vi "Multirecord Acquisition FPGA_20221228.vi"() -> ()   [LabVIEW 2021]
doc: "Use this VI as a template for the reconfigurable oscilloscope acquisition design. The block diagram is divided into three main loops.\n\nRegister Bus: This loop initializes the registers that are needed to support the configuration of the device. The FIFO bus, on the left, allows all the other design libraries to communicate with one another. This loop is very important to support the proper behavior of the instrument design library components.\n\nAcquisition: Acquires data from the I/O channels and writes the data into the record memory using the <B>Write</B> VI of the Multirecord Acquisition instrument design library. This VI also evaluates the various acquisition triggers and decides whether to acquire each data value in record memory. The host level VI (Fetch Record.vi) can read acquired records from the DRAM. The data is stored in 2 DRAM banks, each with 768 MB of storage.\n\nFetch: The recorded data is retrieved when the <B>Fetch Single Record</B> VI is run from the host VI. The <B>Write to Fetch DMA FIFO</B> VI writes data to the acq.fetch fifo 0 to transmit record data form the FPGA to the record fetch VIs on the host. This DMA FIFO must have a predefined name based on the instance parameter. By default, it is 0 (since the associated terminal on the <B>Create Resources DRAM Write Read</B> VI is unwired), so the connected FIFO is named acq.fetch fifo 0."
uses:
  FPGA Interface Typedefinitions/Trigger Combination Type.ctl
  Host/Clusts/AllWindowsClust.ctl
  Host/Clusts/ChannelWindowClust.ctl
  Controls/Clust/WindowTriggerClust.ctl
  <instrlib>/_niInstr/Data Trigger/v1/Shared/Public/Level Configuration FXP(+-,18,1).ctl
  <instrlib>/_niInstr/Data Trigger/v1/Shared/Public/Level Configuration Trigger When.ctl
  <vilib>/Platform/TimedLoop/XDataNode/timing_clust.ctl
  <vilib>/Platform/TimedLoop/XDataNode/nitl_modes.ctl
  <vilib>/Platform/TimedLoop/XDataNode/wakeup.ctl
  Controls/Clust/All_acquisition_Resources.ctl
  <instrlib>/_niInstr/Multirecord Acquisition/Common/v1/FPGA/niInstr Multirecord Acquisition Common v1 FPGA.lvclass
  C:/Program Files (x86)/National Instruments/LabVIEW 2021/instr.lib/_niInstr/Multirecord Acquisition/Interface/v1/FPGA/niInstr Multirecord Acquisition v1 FPGA.lvclass
  Trigger/SubVIs/Types/Trigger Type.ctl
  <instrlib>/_niInstr/Data Trigger/v1/Shared/Public/Edge Configuration FXP(+-,18,1).ctl
  <instrlib>/_niInstr/Data Trigger/v1/Shared/Public/Edge Configuration Trigger Slope.ctl
  Controls/Clust/Update_Trigger_Center.ctl
  Controls/Clust/Status_Booleans_Clust.ctl
  Controls/Clust/Trig_Config_Clust.ctl
  <instrlib>/_niInstr/FIFO Register Bus/v1/FPGA/niInstr FIFO Register Bus v1 FPGA.lvclass
  C:/Program Files (x86)/National Instruments/LabVIEW 2021/instr.lib/_niInstr/Instruction Framework/v1/FPGA/Interfaces/Instruction Producer/Instruction Producer.lvclass
  <vilib>/rvi/Emulation/niFpgaSctlEmulationGetInTimedLoop.vi
  <vilib>/rvi/Emulation/niFpgaEmulationReportErrorSimple.vi
  <vilib>/rvi/Emulation/niFpgaGetClockAttributes.vi
  <vilib>/rvi/Emulation/niFpgaCriticalErrorInLSC.vi
  <instrlib>/_niInstr/Multirecord Acquisition/Common/v1/FPGA/Private/Create Fetch DMA FIFO Resources U8x32.vi
  <instrlib>/_niInstr/Multirecord Acquisition/Common/v1/FPGA/Private/Create Resources DRAM U384x2 U768 Write Read.vi
  <instrlib>/_niInstr/Basic Elements/v1/FPGA/Private/Count Up U32.vi
  <vilib>/rvi/eio/common/nirviEmuTemplateMethod_errors.vi
  <instrlib>/HSAI-RIO/Config/Group A/v1/FPGA/Digital Correction/Validate 8 Channel Data.vi
  <instrlib>/HSAI-RIO/Config/Group A/v1/FPGA/Digital Correction/Digital Correction (8 Ch).vi
  <instrlib>/HSAI-RIO/Config/Group A/v1/FPGA/Digital Correction/FIR Filter (8 Ch).vi
  DSP/SubVIs/Integer decimationx8ch.vi
  Data Type Conversion/SubVIs/Remove Overflow FXP(+-,18,1)x8ch.vi
  Trigger/Trigger FXP(+,-,18,1).vi
  Data Type Conversion/SubVIs/Data Type Conversion FXP(+-,18,1) to I16x8ch.vi
  <instrlib>/_niInstr/Channel/v1/FPGA/Private/Select and Interleave/Select And Interleave I16xNspcx8ch.vi
  <instrlib>/_niInstr/Multirecord Acquisition/Interface/v1/FPGA/Private/Write I16 Wrapper.vi
  <instrlib>/_niInstr/Multirecord Acquisition/Interface/v1/FPGA/Private/Retrieve Record U16 Wrapper.vi
  <instrlib>/_niInstr/Multirecord Acquisition/Interface/v1/FPGA/Private/Write to Fetch DMA FIFO U16 Wrapper.vi
  <vilib>/Platform/TimedLoop/XDataNode/XDataNode.xnode
  <vilib>/eio/EIONode/EIONode.xnode
  <instrlib>/_niInstr/Instruction Framework/v1/FPGA/Top Level Bus/Register Configuration/Register Configuration.lvclass
  <vilib>/Platform/TimedLoop/XDataNode/XDNodeRunTimeDep.lvlib
  <instrlib>/_niInstr/Multirecord Acquisition/Interface/v1/FPGA/niInstr Multirecord Acquisition v1 FPGA.lvclass
  <vilib>/rvi/LocalResourceManager/LocalResourceManager.xnode
  <vilib>/rvi/eio/common/nirviEmuReportErrorAndStop.vi
  <vilib>/rvi/DataTransferAndStorage/Container/Common/niFpgaContainerGetUniqueNameForEmu.vi
  <vilib>/rvi/DataTransferAndStorage/Container/Common/niFpgaContainerSetEmuInfo.vi
  <instrlib>/_niInstr/Channel/v1/FPGA/niInstr Channel v1 FPGA.lvlib
  <instrlib>/_niInstr/Basic Elements/v1/FPGA/niInstr Basic Elements v1 FPGA.lvlib
  <instrlib>/HSAI-RIO/Config/Group A/v1/FPGA/Digital Correction/Digital Correction.lvclass
  <instrlib>/HSAI-RIO/Config/Group A/v1/FPGA/Config Registers/Config Registers.lvclass
  <instrlib>/_niInstr/Data Trigger/v1/Shared/niInstr Data Trigger v1 Shared.lvlib
  Emulation/SubVIs/2 Element Generate Sine Cos Data FXP(+,-,14,1).vi
  <instrlib>/_niInstr/Multirecord Acquisition/Common/v1/FPGA/Private/Create Resources DRAM U384.vi
  <instrlib>/_niInstr/Multirecord Acquisition/Common/v1/FPGA/Private/Create Resources BRAM U384.vi
  <instrlib>/_niInstr/Multirecord Acquisition/Common/v1/FPGA/Private/Create Resources BRAM U768.vi
  FPGA Interface Typedefinitions/FPGA Interface Typedefinitions.lvlib
  C:/Program Files (x86)/National Instruments/LabVIEW 2021/instr.lib/_niInstr/Multirecord Acquisition/Common/v1/FPGA/niInstr Multirecord Acquisition Common v1 FPGA.lvclass
panel:
  out "Trigger Index":u16
  out "TrigCount":u32
  out "TrigCfg 0":T1
  in  "ResetTrig":bool
  in  "UserTrig":T4
  in  "trigger.rearm delay":u16=2
  in  "start trigger":bool=TRUE
  in  "reset":bool
  in  "trigger.combination type":T6
  out "fifo reg bus data 0":u64
  out "fifo reg bus status 0":u32
  in  "fifo reg bus ctrl 0":u32
  out "overflow":bool
  in  "dsp.decimation factor":u16
  out "overload":bool
  # "Register Bus Controls"
  # "FPGA"
  # "Acquisition Loop Controls"
  # "DSP"
  # "Trigger"
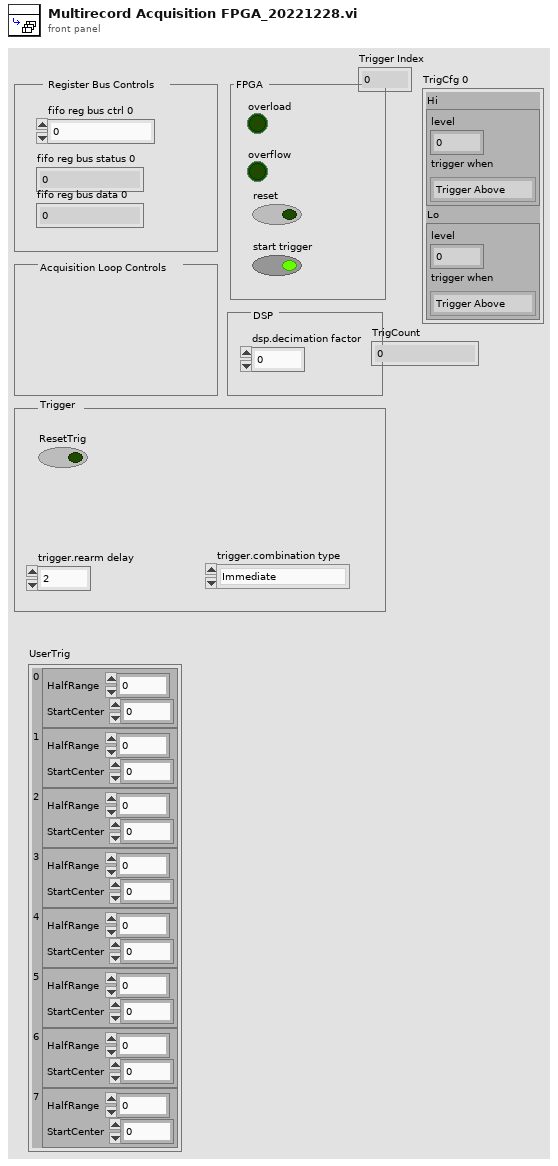
[diagram p1: front panel]
types:
  T1 = typedef "WindowTriggerClust.ctl" = cluster{"Hi":T2, "Lo":T2}
  T2 = typedef "niInstr Data Trigger v1 Shared.lvlib/Level Configuration FXP(+-,18,1).ctl" = cluster{"level":fxp<+/-,18,5>, "trigger when":T3}
  T3 = typedef "niInstr Data Trigger v1 Shared.lvlib/Level Configuration Trigger When.ctl" = enum8{"Trigger Above", "Trigger Below"}
  T4 = typedef "AllWindowsClust.ctl" = cluster{"0":T5, "1":T5, "2":T5, "3":T5, "4":T5, "5":T5, "6":T5, "7":T5}
  T5 = typedef "ChannelWindowClust.ctl" = cluster{"HalfRange":fxp<+/-,18,5>, "StartCenter":fxp<+/-,18,5>}
  T6 = typedef "FPGA Interface Typedefinitions.lvlib/Trigger Combination Type.ctl" = enum16{"Immediate", "A", "B", "OR", "AND", "A THEN B", "B THEN A", "High Resolution"}
  T7 = typedef "All_acquisition_Resources.ctl" = cluster{"acquisition resources 0":refnum<class "niInstr Multirecord Acquisition Common v1 FPGA.lvclass">, "acquisition resources 1":refnum<class "niInstr Multirecord Acquisition Common v1 FPGA.lvclass">, "acquisition resources 2":refnum<class "niInstr Multirecord Acquisition Common v1 FPGA.lvclass">, "acquisition resources 3":refnum<class "niInstr Multirecord Acquisition Common v1 FPGA.lvclass">, "acquisition resources 4":refnum<class "niInstr Multirecord Acquisition Common v1 FPGA.lvclass">, "acquisition resources 5":refnum<class "niInstr Multirecord Acquisition Common v1 FPGA.lvclass">, "acquisition resources 6":refnum<class "niInstr Multirecord Acquisition Common v1 FPGA.lvclass">, "acquisition resources 7":refnum<class "niInstr Multirecord Acquisition Common v1 FPGA.lvclass">}
  T8 = cluster{"memory 1":refnum<k21>, "memory 2":refnum<k21>}
  T9 = typedef "XDNodeRunTimeDep.lvlib/timing_clust.ctl" = cluster{"Expected End [f-1]":u64, "Actual End [f-1]":u64, "Finished Late? [f-1]":bool, "Expected End [i-1]":u64, "Actual End [i-1]":u64, "Finished Late? [i-1]":bool, "Expected Start [i]":u64, "Actual Start [i]":u64, "Expected Start [f]":u64, "Actual Start [f]":u64, "Source Name":string, "Structure Name":string, "Period":i64, "Deadline":i64, "Offset":i64, "Start":i64, "Priority":i32, "Timeout":i32, "Mode":T10, "Wakeup Reason":T11, "Error":errorcluster, "Source Type":string, "Secondary Source Type":string, "Global End Time":u64, "Global Start Time":u64, "Frame Duration":u64, "Iteration Duration":u64, "Assigned CPU":i32, "I/O Scan Engine Mode":u32}
  T10 = typedef "XDNodeRunTimeDep.lvlib/nitl_modes.ctl" = enum32{"No Change", "Process missed periods, maintain original phase", "Discard missed periods, maintain original phase", "Process missed periods, ignore original phase", "Discard missed periods, ignore original phase"}
  T11 = typedef "XDNodeRunTimeDep.lvlib/wakeup.ctl" = enum32{"Normal", "Aborted", "Asynchronous wakeup", "Timing source error", "Timed loop error", "Timeout"}
  T12 = typedef "Trig_Config_Clust.ctl" = cluster{"UserTrig":T4, "type":T6, "rearm delay":u16}
  T13 = typedef "Status_Booleans_Clust.ctl" = cluster{"reset out":bool, "ResetTrig":bool, "output valid":bool}
  T14 = typedef "Update_Trigger_Center.ctl" = cluster{"New Center":fxp<+/-,18,5>, "apply":bool}
  T15 = typedef "Trigger Type.ctl" = enum16{"Edge", "Level", "Custom"}
  T16 = typedef "niInstr Data Trigger v1 Shared.lvlib/Edge Configuration FXP(+-,18,1).ctl" = cluster{"highLevel":fxp<+/-,18,1>, "lowLevel":fxp<+/-,18,1>, "trigger slope":T17}
  T17 = typedef "niInstr Data Trigger v1 Shared.lvlib/Edge Configuration Trigger Slope.ctl" = enum8{"Positive", "Negative"}
  T18 = cluster{"Channel 0":fxp<+/-,14,1>[], "Channel 1":fxp<+/-,14,1>[], "Channel 2":fxp<+/-,14,1>[], "Channel 3":fxp<+/-,14,1>[], "Channel 4":fxp<+/-,14,1>[], "Channel 5":fxp<+/-,14,1>[], "Channel 6":fxp<+/-,14,1>[], "Channel 7":fxp<+/-,14,1>[]}
  T19 = cluster{"Channel 0":fxp<+/-,18,1>[], "Channel 1":fxp<+/-,18,1>[], "Channel 2":fxp<+/-,18,1>[], "Channel 3":fxp<+/-,18,1>[], "Channel 4":fxp<+/-,18,1>[], "Channel 5":fxp<+/-,18,1>[], "Channel 6":fxp<+/-,18,1>[], "Channel 7":fxp<+/-,18,1>[]}
  T20 = cluster{"channel 0":fxp<+/-,18,1>[], "channel 1":fxp<+/-,18,1>[], "channel 2":fxp<+/-,18,1>[], "channel 3":fxp<+/-,18,1>[], "channel 4":fxp<+/-,18,1>[], "channel 5":fxp<+/-,18,1>[], "channel 6":fxp<+/-,18,1>[], "channel 7":fxp<+/-,18,1>[]}
  T21 = cluster{"channel 0":i16[], "channel 1":i16[], "channel 2":i16[], "channel 3":i16[], "channel 4":i16[], "channel 5":i16[], "channel 6":i16[], "channel 7":i16[]}
  T22 = typedef "niInstr Multirecord Acquisition v1 FPGA.lvclass/Timestamp.ctl" = cluster{"timestamp":u64, "valid":bool}
  T23 = typedef "niInstr Types v1 Shared.lvlib/Input Triggers.ctl" = cluster{"start":bool, "advance":bool, "reference":bool, "start trigger index":u16, "advance trigger index":u16, "reference trigger index":u16, "reference trigger correction cycle count":u32}
  T24 = typedef "niInstr Types v1 Shared.lvlib/Sample Format.ctl" = cluster{"bits per channel":u16, "samples per clock":u16, "channels":u8}
  T25 = typedef "niInstr Multirecord Acquisition v1 FPGA.lvclass/Events.ctl" = cluster{"ready for start":bool, "ready for advance":bool, "ready for reference":bool, "end of record":bool, "done":bool, "start trigger":bool, "advance trigger":bool, "reference trigger":bool, "start trigger index":u16, "advance trigger index":u16, "reference trigger index":u16}
  T26 = typedef "All_Window_Triggers_Clust.ctl" = cluster{"0":T1, "1":T1, "2":T1, "3":T1, "4":T1, "5":T1, "6":T1, "7":T1}
  T27 = typedef "niInstr Multirecord Acquisition v1 FPGA.lvclass/Retrieve Data Info.ctl" = cluster{"read request size (bits)":u64, "valid data offset (bits)":u16, "valid data size (bits)":u16, "first sample of request":bool, "last sample of request":bool, "Token":T28}
  T28 = typedef "niInstr Types v1 Shared.lvlib/Token.ctl" = cluster{"identifier":u8, "value":u32}
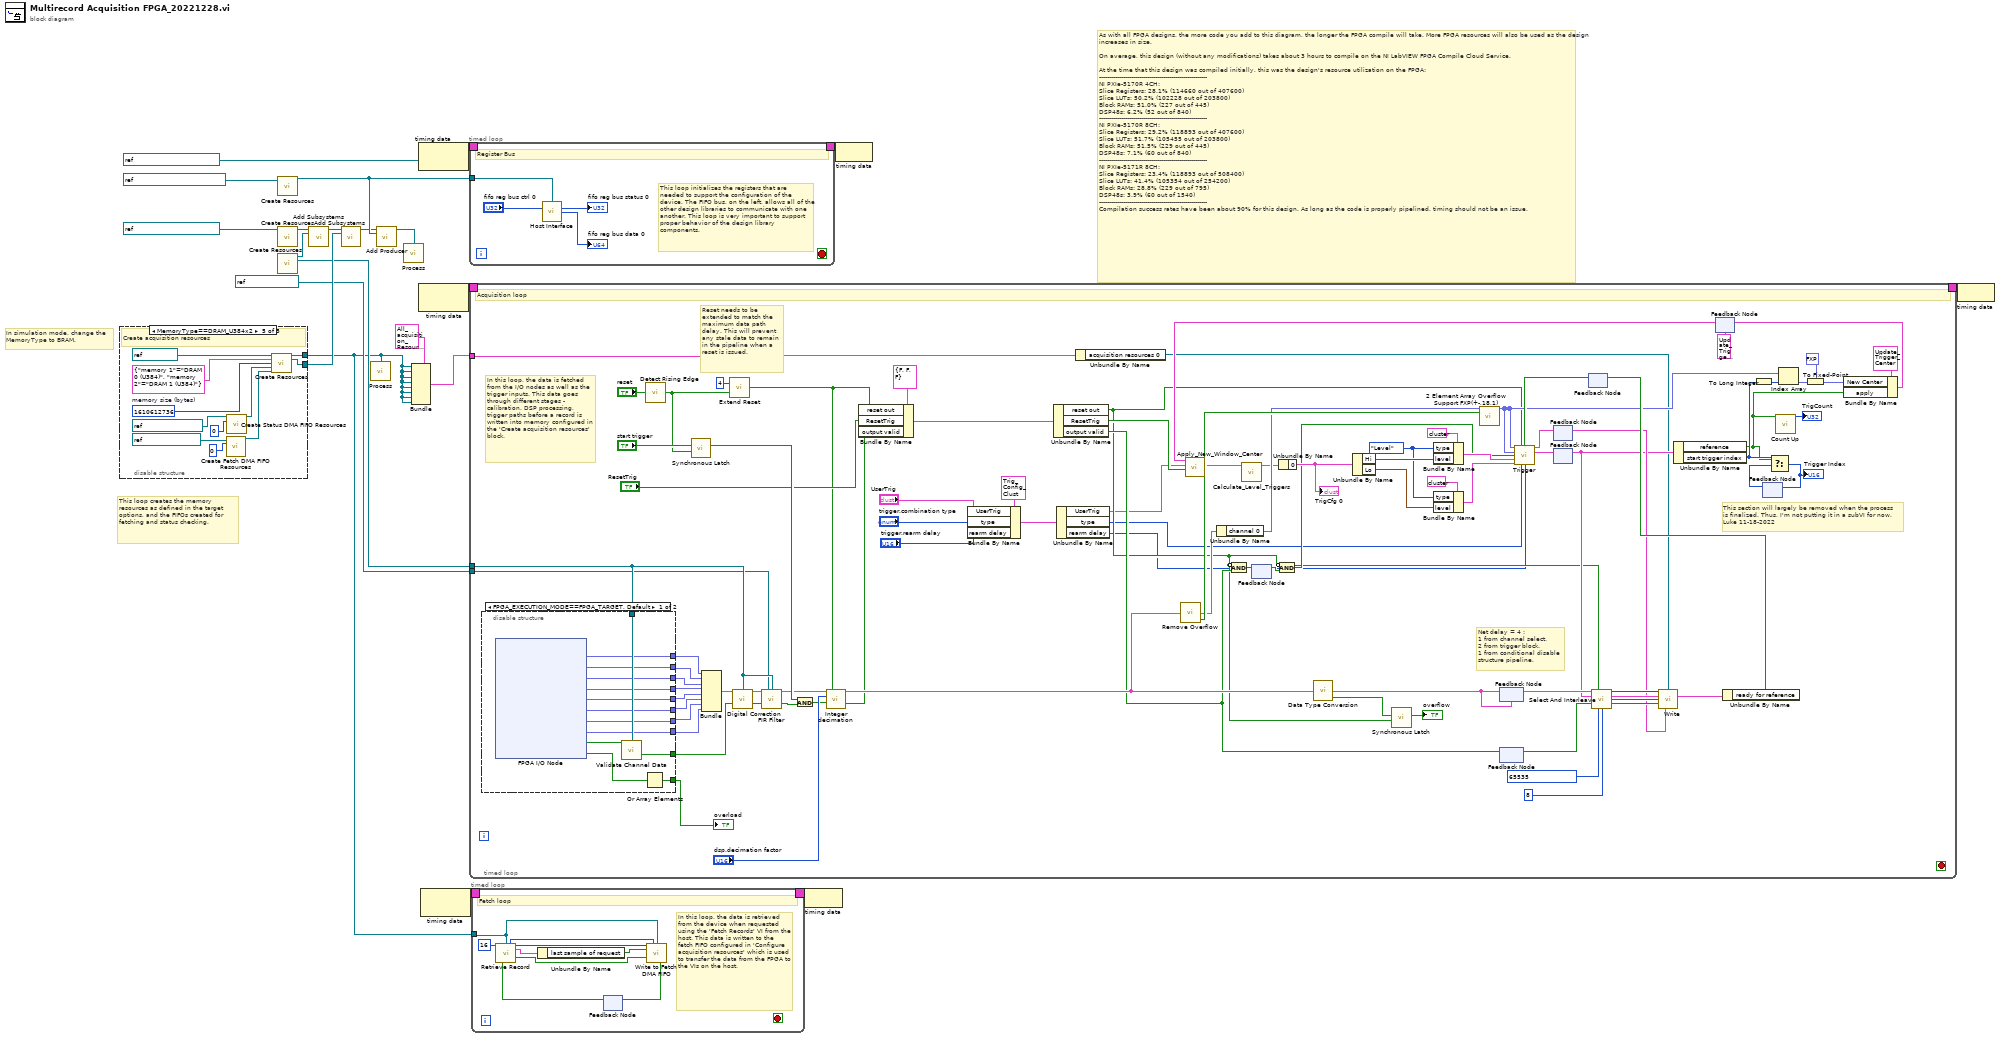
[diagram p0: block diagram]
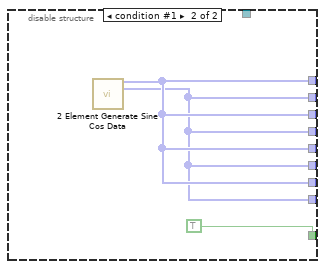
[diagram p2: hidden frame]
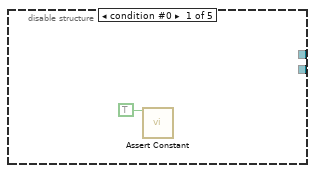
[diagram p3: hidden frame]
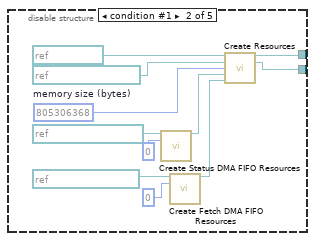
[diagram p4: hidden frame]
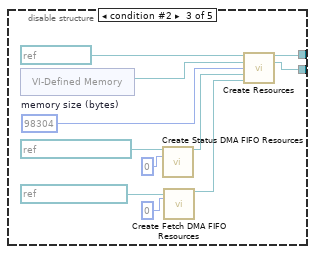
[diagram p5: hidden frame]
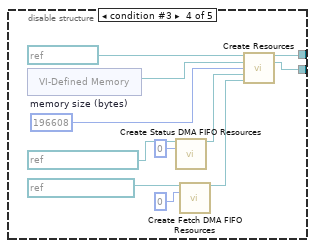
[diagram p6: hidden frame]
diagram:
  # "In simulation mode, change the MemoryType to BRAM."
  # "This loop creates the memory resources as defined in the target options, and the FIFOs created for fetching and status checking."
  # "As with all FPGA designs, the more code you add to this diagram, the longer the FPGA compile will take. More FPGA resources will also be used as the design increases in size.\n\nOn average, this design (without any modifications) takes about 3 hours to compile on the NI LabVIEW FPGA Compile Cloud Service. \n\nAt the time that this design was compiled initially, this was the design's resource utilization on the FPGA:\n------------------------------------------------------\nNI PXIe-5170R 4CH:\nSlice Registers: 28.1% (114660 out of 407600)\nSlice LUTs: 50.2% (102228 out of 203800)\nBlock RAMs: 51.0% (227 out of 445)\nDSP48s: 6.2% (52 out of 840)\n------------------------------------------------------\nNI PXIe-5170R 8CH:\nSlice Registers: 29.2% (118893 out of 407600)\nSlice LUTs: 51.7% (105455 out of 203800)\nBlock RAMs: 51.5% (229 out of 445)\nDSP48s: 7.1% (60 out of 840)\n------------------------------------------------------\nNI PXIe-5171R 8CH:\nSlice Registers: 23.4% (118893 out of 508400)\nSlice LUTs: 41.4% (105354 out of 254200)\nBlock RAMs: 28.8% (229 out of 795)\nDSP48s: 3.9% (60 out of 1540)\n------------------------------------------------------\nCompilation success rates have been about 90% for this design. As long as the code is properly pipelined, timing should not be an issue."
  n1 = disable-structure shown="MemoryType==DRAM_U384x2" {
    disable-tunnel: [_ w31 w42 w53 w64] -> w2
    disable-tunnel: [_ w28 w38 w49 w61] -> w9
    frame condition #0 {
      n2 = call <instrlib>:"Assert Constant.vi"("constant terminal"=TRUE) -> ()  [unwired: 15 in]
    }
    frame condition #1 {
      w32 = u64 805306368  # memory size (bytes)
      n3 = call <instrlib>:"Create Status DMA FIFO Resources.vi"("status dma fifo in"=refnum<k21> "acq.status fifo 0" ("status dma fifo"), "fifo instance"=u8 0) -> ("status dma fifo out"=w23:refnum<class "niInstr Status FIFO v1 FPGA.lvclass">)  [unwired: 13 in]
      n4 = call-poly <instrlib>:"Create Fetch DMA FIFO Resources.vi"("fetch dma fifo in"=refnum<k21> "acq.fetch fifo 0", "fifo instance"=u8 0) -> ("fetch dma fifo out"=w29:refnum<class "niInstr Fetch FIFO v1 FPGA.lvclass">)  [unwired: 13 in]
      n5 = call-poly <instrlib>:"Create Resources.vi"("memory clock"=refnum<k21> "160MHz" ("process clock"), "memory"=refnum<k21> "DRAM 0 (U384)" ("dram"), "memory size (bytes)"=w32, "status dma fifo resources"=w23, "fetch dma fifo resources"=w29) -> ("acquisition resources"=w31:refnum<class "niInstr Multirecord Acquisition Common v1 FPGA.lvclass">, "acquisition subsystem"=w28:refnum<class "Address Space Collection.lvclass">)  [unwired: 9 in]
    }
    frame condition #2 {
      w43 = u64 98304  # memory size (bytes)
      n6 = xnode "VI-Defined Memory"() -> ("Memory Out"=w44:refnum<k21>)
      n7 = call <instrlib>:"Create Status DMA FIFO Resources.vi"("status dma fifo in"=refnum<k21> "acq.status fifo 0" ("status dma fifo"), "fifo instance"=u8 0) -> ("status dma fifo out"=w35:refnum<class "niInstr Status FIFO v1 FPGA.lvclass">)  [unwired: 13 in]
      n8 = call-poly <instrlib>:"Create Fetch DMA FIFO Resources.vi"("fetch dma fifo in"=refnum<k21> "acq.fetch fifo 0", "fifo instance"=u8 0) -> ("fetch dma fifo out"=w39:refnum<class "niInstr Fetch FIFO v1 FPGA.lvclass">)  [unwired: 13 in]
      n9 = call-poly <instrlib>:"Create Resources.vi"("memory clock"=refnum<k21> "160MHz" ("process clock"), "memory"=w44, "memory size (bytes)"=w43, "status dma fifo resources"=w35, "fetch dma fifo resources"=w39) -> ("acquisition resources"=w42:refnum<class "niInstr Multirecord Acquisition Common v1 FPGA.lvclass">, "acquisition subsystem"=w38:refnum<class "Address Space Collection.lvclass">)  [unwired: 9 in]
    }
    frame condition #3 {
      w54 = u64 196608  # memory size (bytes)
      n10 = xnode "VI-Defined Memory"() -> ("Memory Out"=w55:refnum<k21>)
      n11 = call <instrlib>:"Create Status DMA FIFO Resources.vi"("status dma fifo in"=refnum<k21> "acq.status fifo 0" ("status dma fifo"), "fifo instance"=u8 0) -> ("status dma fifo out"=w47:refnum<class "niInstr Status FIFO v1 FPGA.lvclass">)  [unwired: 13 in]
      n12 = call-poly <instrlib>:"Create Fetch DMA FIFO Resources.vi"("fetch dma fifo in"=refnum<k21> "acq.fetch fifo 0", "fifo instance"=u8 0) -> ("fetch dma fifo out"=w50:refnum<class "niInstr Fetch FIFO v1 FPGA.lvclass">)  [unwired: 13 in]
      n13 = call-poly <instrlib>:"Create Resources.vi"("memory clock"=refnum<k21> "160MHz" ("process clock"), "memory"=w55, "memory size (bytes)"=w54, "status dma fifo resources"=w47, "fetch dma fifo resources"=w50) -> ("acquisition resources"=w53:refnum<class "niInstr Multirecord Acquisition Common v1 FPGA.lvclass">, "acquisition subsystem"=w49:refnum<class "Address Space Collection.lvclass">)  [unwired: 9 in]
    }
    frame condition #4 (active) {
      w66 = u64 1610612736  # memory size (bytes)
      # "Create acquisition resources"
      n14 = call-poly <instrlib>:"Create Fetch DMA FIFO Resources.vi"("fetch dma fifo in"=refnum<k21> "acq.fetch fifo 0", "fifo instance"=u8 0) -> ("fetch dma fifo out"=w63:refnum<class "niInstr Fetch FIFO v1 FPGA.lvclass">)  [unwired: 13 in]
      n15 = call <instrlib>:"Create Status DMA FIFO Resources.vi"("status dma fifo in"=refnum<k21> "acq.status fifo 0" ("status dma fifo"), "fifo instance"=u8 0) -> ("status dma fifo out"=w58:refnum<class "niInstr Status FIFO v1 FPGA.lvclass">)  [unwired: 13 in]
      n16 = call-poly <instrlib>:"Create Resources.vi"("memory clock"=refnum<k21> "160MHz" ("process clock"), "memory"=T8 {"memory 1"="DRAM 0 (U384)", "memory 2"="DRAM 1 (U384)"}, "memory size (bytes)"=w66, "status dma fifo resources"=w58, "fetch dma fifo resources"=w63) -> ("acquisition resources"=w64:refnum<class "niInstr Multirecord Acquisition Common v1 FPGA.lvclass">, "acquisition subsystem"=w61:refnum<class "Address Space Collection.lvclass">)  [unwired: 9 in]
    }
  }
  n17 = call <instrlib>:"Create Resources.vi"("instruction fifo"=refnum<k21> "reg.host instruction fifo 0" ("FIFO")) -> ("fifo register bus"=w8:refnum<class "niInstr FIFO Register Bus v1 FPGA.lvclass">)  [unwired: 14 in]
  n18 = call <instrlib>:"Create Resources.vi"("register clock"=refnum<k21> "40 MHz Onboard Clock" ("Source Name")) -> ("register configuration"=w12:refnum<class "Register Configuration.lvclass">)  [unwired: 14 in]
  n19 = call <instrlib>:"Create Resources.vi"() -> ("config subsystems"=w10:refnum<class "Address Space Collection.lvclass">, "digital correction resources"=w4:refnum<class "Digital Correction.lvclass">)  [unwired: 14 in]
  n20 = call-dynamic "Add Subsystems.vi"("register configuration in"=w12, "subsystems"=w10) -> ("register configuration out"=w11:refnum<class "Register Configuration.lvclass">)  [unwired: 13 in]
  n21 = call-dynamic "Add Subsystems.vi"("register configuration in"=w11, "subsystems"=w9) -> ("register configuration out"=w6:refnum<class "Register Configuration.lvclass">)  [unwired: 13 in]
  n22 = call-dynamic "Process.vi"("acquisition resources"=w2) -> ()  [unwired: 15 in]
  n23 = call-dynamic "Add Producer.vi"("register configuration in"=w6, "instruction producer"=w8) -> ("register configuration out"=w7:refnum<class "Register Configuration.lvclass">)  [unwired: 13 in]
  n24 = call-dynamic "Process.vi"("register configuration"=w7) -> ()  [unwired: 15 in]
  n25 = Bundle(cluster=T7 {"acquisition resources 0"=refnum, "acquisition resources 1"=refnum, "acquisition resources 2"=refnum, "acquisition resources 3"=refnum, "acquisition resources 4"=refnum, "acquisition resources 5"=refnum, "acquisition resources 6"=refnum, "acquisition resources 7"=refnum}, "acquisition resources 0"=w2, "acquisition resources 1"=w2, "acquisition resources 2"=w2, "acquisition resources 3"=w2, "acquisition resources 4"=w2, "acquisition resources 5"=w2, "acquisition resources 6"=w2, "acquisition resources 7"=w2) -> (w1:T7)
  n26 = node-c288(refnum<k21> "40 MHz Onboard Clock" ("Source Name")) -> (w21:T9)
  n27 = node-c288() -> (w19:T9)  [unwired: 1 in]
  n28 = node-c288() -> (w17:T9)  [unwired: 1 in]
  n29 = timed-loop {
    timing: w21 -> [_]
    timing-out: [_] -> w20
    tunnel: w8 -> [w70]
    stop <- _ stop-if-true
    # "This loop initializes the registers that are needed to support the configuration of the device. The FIFO bus, on the left, allows all of the other design libraries to communicate with one another. This loop is very important to support proper behavior of the design library components."
    # "Register Bus"
    n30 = call <instrlib>:"Host Interface.vi"("fifo register bus"=w70, "fifo reg bus ctrl 0"="fifo reg bus ctrl 0") -> ("fifo reg bus status 0"=→"fifo reg bus status 0":u32, "fifo reg bus data 0"=→"fifo reg bus data 0":u64)  [unwired: 12 in]
  }
  n31 = timed-loop {
    timing: w19 -> [_]
    timing-out: [_] -> w18
    tunnel: w1 -> [w73]
    tunnel: w4 -> [w141]
    tunnel: refnum<k21> "Data Clock x2" -> [w138]
    stop <- _ stop-if-true
    w135 = Trigger_Type."Level" ("type")
    # "This section will largely be removed when the process\nis finalized. Thus, I'm not putting it in a subVI for now.\nLuke 11-18-2022"
    # "Net delay = 4 :\n1 from channel select.\n2 from trigger block.\n1 from conditional disable structure pipeline."
    # "Reset needs to be extended to match the maximum data path delay. This will prevent any stale data to remain in the pipeline when a reset is issued."
    # "In this loop, the data is fetched from the I/O nodes as well as the trigger inputs. This data goes through different stages - calibration, DSP processing, trigger paths before a record is written into memory configured in the 'Create acquisition resources' block."
    # "Acquisition loop"
    n32 = disable-structure shown="FPGA_EXECUTION_MODE==FPGA_TARGET, Default" {
      disable-tunnel: [w174 w179] -> w127
      disable-tunnel: [w173 w178] -> w126
      disable-tunnel: [w172 w179] -> w125
      disable-tunnel: [w171 w178] -> w124
      disable-tunnel: [w170 w179] -> w123
      disable-tunnel: [w169 w178] -> w122
      disable-tunnel: [w168 w179] -> w120
      disable-tunnel: [w167 w178] -> w121
      disable-tunnel: [w164 TRUE ("ADC Data Valid")] -> w118
      disable-tunnel: w141 -> [w175 _]
      disable-tunnel: [w165 _] -> w162
      frame condition #0 (active) {
        # "I/O Nodes"
        n33 = xnode "FPGA I/O Node"() -> ("Channel 0"=w174:fxp<+/-,14,1>[], "Channel 1"=w173:fxp<+/-,14,1>[], "Channel 2"=w172:fxp<+/-,14,1>[], "Channel 3"=w171:fxp<+/-,14,1>[], "Channel 4"=w170:fxp<+/-,14,1>[], "Channel 5"=w169:fxp<+/-,14,1>[], "Channel 6"=w168:fxp<+/-,14,1>[], "Channel 7"=w167:fxp<+/-,14,1>[], "Channel Data Valid"=w176:bool[], "Channel Overload"=w166:bool[])  [unwired: 10 in, 10 out]
        n34 = call-poly <instrlib>:"Validate Channel Data.vi"("channel data valid"=w176, "digital correction resources"=w175) -> ("expected data valid"=w164:bool)  [unwired: 13 in]
        n35 = Or Array Elements(Boolean array=w166) -> (logical OR=w165:bool)
      }
      frame condition #1 {
        n36 = call-poly "2 Element Generate Sine Cos Data.vi"() -> ("sine data"=w179:fxp<+/-,14,1>[], "cosine data"=w178:fxp<+/-,14,1>[])  [unwired: 14 in]
      }
    }
    "overload" <- w162
    n37 = call <instrlib>:"Detect Rising Edge.vi"("signal"="reset") -> ("edge detected"=w140:bool)  [unwired: 14 in]
    n38 = call <instrlib>:"Synchronous Latch.vi"("clear"=w140, "set"="start trigger") -> ("out"=w145:bool)  [unwired: 9 in]
    n39 = Bundle("Channel 0"=w127, "Channel 1"=w126, "Channel 2"=w125, "Channel 3"=w124, "Channel 4"=w123, "Channel 5"=w122, "Channel 6"=w120, "Channel 7"=w121) -> (w119:T18)  [unwired: 1 in]
    n40 = call "Extend Reset.vi"("reset in"=w140, "number of cycles"=u8 4) -> ("reset out"=w84:bool)
    n41 = call-poly <instrlib>:"Digital Correction.vi"("channel data in"=w119, "digital correction resources"=w141, "input valid"=w118) -> ("corrected channel data out"=w111:T19, "output valid"=w110:bool)  [unwired: 11 in]
    n42 = call-poly <instrlib>:"FIR Filter.vi"("data in"=w111, "data clock x2"=w138, "digital correction resources"=w141, "input valid"=w110) -> ("data out"=w108:T19, "output valid"=w109:bool)  [unwired: 9 in, 1 out]
    n43 = And(x=w145, y=w109) -> (x .and. y?=w112:bool)
    n44 = call-poly "Integer decimation.vi"("data in"=w108, "reset"=w84, "decimation factor"="dsp.decimation factor", "input valid"=w112) -> ("data out"=w115:T20, "output valid"=w86:bool)  [unwired: 9 in, 1 out]
    n45 = Bundle By Name(cluster=T13 {"reset out"=FALSE, "ResetTrig"=FALSE, "output valid"=FALSE} ("Status"), "reset out"=w84, "ResetTrig"="ResetTrig", "output valid"=w86) -> (w89:T13)
    n46 = Bundle By Name(cluster=T12 {"UserTrig"={"0"={"HalfRange"=0.0, "StartCenter"=0.0}, "1"={"HalfRange"=0.0, "StartCenter"=0.0}, "2"={"HalfRange"=0.0, "StartCenter"=0.0}, "3"={"HalfRange"=0.0, "StartCenter"=0.0}, "4"={"HalfRange"=0.0, "StartCenter"=0.0}, "5"={"HalfRange"=0.0, "StartCenter"=0.0}, "6"={"HalfRange"=0.0, "StartCenter"=0.0}, "7"={"HalfRange"=0.0, "StartCenter"=0.0}}, "type"=enum."Immediate", "rearm delay"=0} ("output cluster"), "UserTrig"="UserTrig", "type"="trigger.combination type", "rearm delay"="trigger.rearm delay") -> (w81:T12)
    n47 = Unbundle By Name(w89) -> ("reset out"=w83:bool, "ResetTrig"=w87:bool, "output valid"=w85:bool)
    n48 = Unbundle By Name(w81) -> ("UserTrig"=w79:T4, "type"=w77:T6, "rearm delay"=w75:u16)
    n49 = Unbundle By Name(w73) -> ("acquisition resources 0"=w74:refnum<class "niInstr Multirecord Acquisition Common v1 FPGA.lvclass">)
    n50 = call-poly "Remove Overflow.vi"("data in"=w115) -> ("overflow"=w147:bool, "data out"=w129:T20)  [unwired: 3 in]
    n51 = Unbundle By Name(w129) -> ("channel 0"=w128:fxp<+/-,18,1>[])
    n52 = Compound Arithmetic op=AND(invert w83, w85) -> (w131:bool)
    n53 = feedback #1() -> (w132:bool)  [unwired: 1 in]
    n54 = feedback-in #1(w131) -> ()
    n55 = Compound Arithmetic op=AND(invert w83, w132) -> (w130:bool)
    n56 = call-poly "Data Type Conversion.vi"("data in"=w115) -> ("overflow"=w117:bool, "data out"=w114:T21)  [unwired: 3 in]
    n57 = call <instrlib>:"Synchronous Latch.vi"("clear"=w83, "set"=w117) -> ("out"=→"overflow":bool)  [unwired: 9 in]
    n58 = call "2 Element Array Overflow Support FXP(+-,18,1).vi"("data in"=w128, "overflow"=w147) -> ("data out"=w103:fxp<+/-,18,1>[])  [unwired: 13 in]
    n59 = feedback #2(w114) -> (w116:T21)
    n60 = feedback-in #2(w114) -> ()
    n61 = feedback #3() -> (w113:bool)  [unwired: 1 in]
    n62 = feedback-in #3(w85) -> ()
    n63 = feedback #4() -> (w133:T22)  [unwired: 1 in]
    n64 = feedback #5() -> (w107:T23)  [unwired: 1 in]
    n65 = feedback #6() -> (w153:bool)  [unwired: 1 in]
    n66 = call-poly <instrlib>:"Select And Interleave.vi"("data in"=w116, "reset"=w83, "triggers in"=w107, "input valid"=w113, "channel enable mask"=u16 65535 ("channel.enable mask"), "number of channels to interleave"=u8 8 ("channel.number of channels")) -> ("interleaved data out"=w161:i16[], "triggers out"=w160:T23, "sample format out"=w159:T24, "output valid"=w158:bool)  [unwired: 5 in, 1 out]
    n67 = call-poly <instrlib>:"Write.vi"("data"=w161, "acquisition resources"=w74, "triggers"=w160, "sample format"=w159, "data valid"=w158, "timestamp"=w133) -> ("events"=w155:T25)  [unwired: 6 in, 3 out]
    n68 = Unbundle By Name(w107) -> ("reference"=w96:bool, "start trigger index"=w102:u16)
    n69 = feedback #7(T14 {"New Center"=0.0, "apply"=FALSE}) -> (w95:T14)
    n70 = call "Apply_New_Window_Center.vi"("ResetTrig"=w87, "User Trig"=w79, "FeedbackTrig"=w95) -> ("AllWindows out"=w91:T4)  [unwired: 8 in]
    n71 = call "Calculate_Level_Triggers.vi"("AllWindows"=w91) -> ("All_Window_Trigs"=w92:T26)  [unwired: 8 in, 2 out]
    n72 = Unbundle By Name(w92) -> ("0"=w137:T1)
    "TrigCfg 0" <- w137
    n73 = Unbundle By Name(w137) -> ("Hi"=w136:T2, "Lo"=w134:T2)
    n74 = Bundle By Name(cluster=cluster{"type":T15, "level":T2, "edge":T16} {"type"=enum."Edge", "level"={"level"=0.0, "trigger when"=enum."Trigger Above"}, "edge"={"highLevel"=0.0, "lowLevel"=0.0, "trigger slope"=enum."Positive"}} ("trigger.A"), "type"=w135, "level"=w136) -> (w149:cluster{"type":T15, "level":T2, "edge":T16})
    n75 = Bundle By Name(cluster=cluster{"type":T15, "level":T2, "edge":T16} {"type"=enum."Edge", "level"={"level"=0.0, "trigger when"=enum."Trigger Above"}, "edge"={"highLevel"=0.0, "lowLevel"=0.0, "trigger slope"=enum."Positive"}} ("trigger.A"), "type"=w135, "level"=w134) -> (w148:cluster{"type":T15, "level":T2, "edge":T16})
    n76 = call-poly "Trigger.vi"("data A"=w103, "reset"=w83, "trigger.ready for reference"=w153, "data B"=w103, "input valid"=w130, "trigger.A"=w149, "trigger.B"=w148, "trigger.combination type"=w77, "rearm delay"=w75) -> ("timestamps"=w143:T22, "trigger.out"=w144:T23)  [unwired: 3 in, 2 out]
    n77 = feedback-in #4(w143) -> ()
    n78 = feedback-in #5(w144) -> ()
    n79 = Unbundle By Name(w155) -> ("ready for reference"=w154:bool)
    n80 = feedback-in #6(w154) -> ()
    n81 = To Long Integer(number=w102) -> (32bit integer=w101:i32)
    n82 = feedback #8() -> (w104:u16)  [unwired: 1 in]
    n83 = Select(t=w102, s=w96, f=w104) -> (s? t:f=w105:u16)
    "Trigger Index" <- w105
    n84 = feedback-in #8(w105) -> ()
    n85 = call-poly <instrlib>:"Count Up.vi"("increment"=w96) -> ("count out"=→"TrigCount":u32)  [unwired: 14 in]
    n86 = Index Array(array=w103, index=w101) -> (element=w100:fxp<+/-,18,1>)
    n87 = To Fixed-Point(fixed-point type=fxp<+/-,18,5> 0.0, number=w100) -> (fixed-point=w97:fxp<+/-,18,5>)
    n88 = Bundle By Name(cluster=T14 {"New Center"=0.0, "apply"=FALSE}, "New Center"=w97, "apply"=w96) -> (w94:T14)
    n89 = feedback-in #7(w94) -> ()
  }
  n90 = timed-loop {
    timing: w17 -> [_]
    timing-out: [_] -> w16
    tunnel: w2 -> [w190]
    stop <- _ stop-if-true
    # "In this loop, the data is retrieved from the device when requested using the 'Fetch Records' VI from the host. This data is written to the fetch FIFO configured in 'Configure acquisition resources' which is used to transfer the data from the FPGA to the VIs on the host."
    # "Fetch loop"
    n91 = feedback #9() -> (w188:bool)  [unwired: 1 in]
    n92 = call-poly <instrlib>:"Retrieve Record.vi"("output array size"=u16 16, "acquisition resources"=w190, "ready for output"=w188) -> ("channels"=w183:u8, "data"=w186:u16[], "retrieve data info"=w185:T27, "output valid"=w187:bool)  [unwired: 9 in]
    n93 = Unbundle By Name(w185) -> ("last sample of request"=w184:bool)
    n94 = call-poly <instrlib>:"Write to Fetch DMA FIFO.vi"("data"=w186, "channels"=w183, "acquisition resources"=w190, "last sample of request"=w184, "input valid"=w187) -> ("ready for input"=w189:bool)  [unwired: 10 in]
    n95 = feedback-in #9(w189) -> ()
  }
  n96 = node-c288(w16) -> ()
  n97 = node-c288(w20) -> ()
  n98 = node-c288(w18) -> ()
